vi "Net test.vi"() -> ()   [LabVIEW 2024]
uses:
  <vilib>/regexp/Match Regular Expression.xnode
panel:
  in  "stop 2":bool
  out "Numeric 2":dbl
  out "Numeric":dbl
  in  "stop":bool
  out "可能的網卡IP位置":string
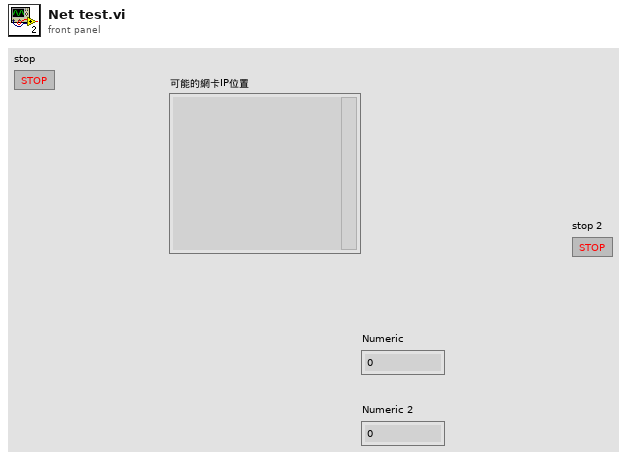
[diagram p1: front panel]
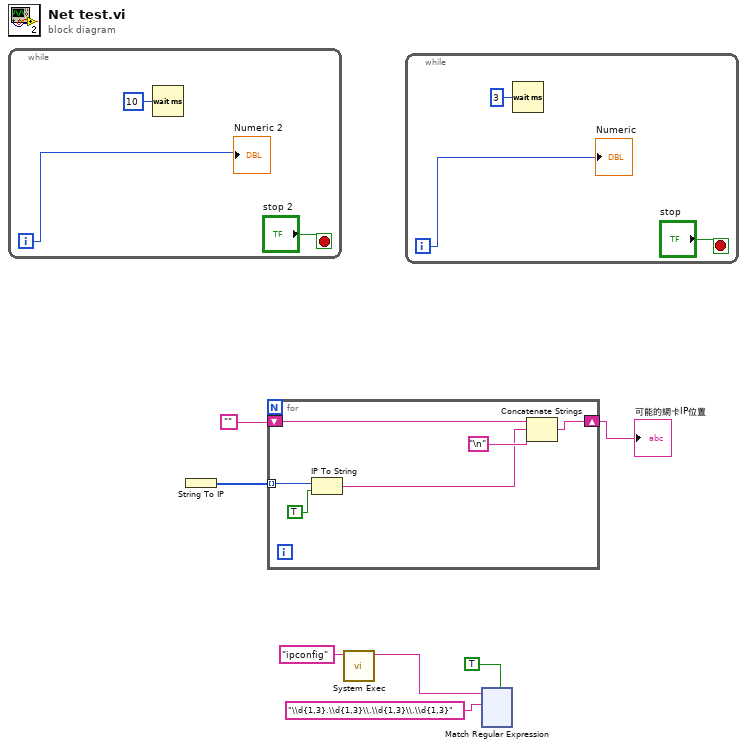
[diagram p0: block diagram]
diagram:
  n1 = while {
    i -> [w9]
    stop <- "stop 2" stop-if-true
    n2 = Wait (ms)(milliseconds to wait=u32 10) -> ()  [unwired: 1 out]
    "Numeric 2" <- w9
  }
  n3 = String To IP() -> (0:w3:u32[])  [unwired: 1 in]
  n4 = for {
    shift-right: [w15] -> w6
    shift-left: "" -> [w16]
    tunnel: w3 -> [w13] mode=indexing
    n5 = IP To String(1:TRUE ("dot notation? (F)"), 2:w13) -> (0:w12:string)
    n6 = Concatenate Strings(w16, w12, "\n") -> (w15:string)
  }
  "可能的網卡IP位置" <- w6
  n7 = call <vilib>:"System Exec.vi"("command line"="ipconfig") -> ("standard output"=w2:string)  [unwired: 7 in, 3 out]
  n8 = while {
    i -> [w18]
    stop <- "stop" stop-if-true
    n9 = Wait (ms)(milliseconds to wait=u32 3) -> ()  [unwired: 1 out]
    "Numeric" <- w18
  }
  n10 = xnode "Match Regular Expression"("input string"=w2, "regular expression"="\\d{1,3}.\\d{1,3}\\.\\d{1,3}\\.\\d{1,3}", "multiline? (F)"=TRUE) -> ()  [unwired: 3 in, 5 out]
